vi "QT_MovieNew.vi"(1 "File Settings":T1 {"Dialogs" format="%.0b"}, 2 "Movie Settings":T4 {"Dialogs" format="%.0b"}, 3 "Compression Settings":T3 {"Dialogs" format="%.0b"; "Comp. Quality" format="%.0x"; "Codec" format="%.0x"}, 5 "error in (no error)":errorcluster, 8 "Private":T5, 9 "Transformation matrix":T2 {"Matrix" format="%.2f"}) -> (14 "QT Ref Out":T6, 19 "error out":errorcluster)   [LabVIEW 2024]
doc: "Create and initilize a new Frame grabber channel"
uses:
  <userlib>/ImageProcessing/QTLIB_2595_LV86/QT_Selector.ctl
  <userlib>/ImageProcessing/QTLIB_2595_LV86/QT_Ref.ctl
  <userlib>/ImageProcessing/QTLIB_2595_LV86/QT_Private.ctl
  <userlib>/ImageProcessing/QTLIB_2595_LV86/QT_Movie.ctl
  <userlib>/ImageProcessing/QTLIB_2595_LV86/QT_Compression.ctl
  <userlib>/ImageProcessing/QTLIB_2595_LV86/QT_File.ctl
  <userlib>/ImageProcessing/QTLIB_2595_LV86/QT_Effect.ctl
panel:
  # "[0,0] [0,1]  [0,2] [1,0].. [2,2]"
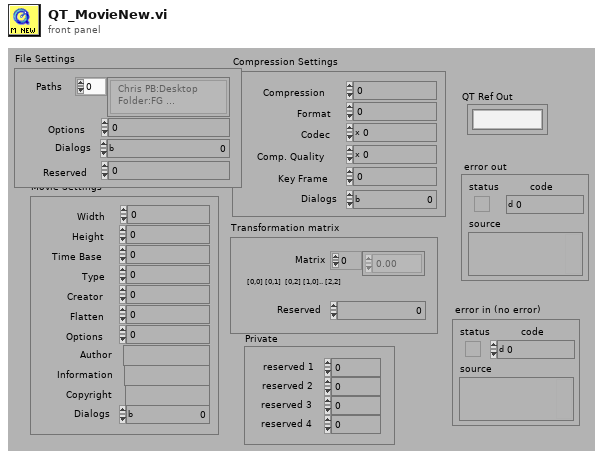
[diagram p1: front panel]
types:
  T1 = typedef "QT_File.ctl" = cluster{"Paths":string[], "Options":i32, "Dialogs":u32, "Reserved":i32}
  T2 = typedef "QT_Effect.ctl" = cluster{"Reserved":i32, "Matrix":dbl[]}
  T3 = typedef "QT_Compression.ctl" = cluster{"Compression":i32, "Format":i32, "Codec":i32, "Comp. Quality":i32, "Key Frame":i32, "Dialogs":u32}
  T4 = typedef "QT_Movie.ctl" = cluster{"Width":i32, "Height":i32, "Time Base":i32, "Type":i32, "Creator":i32, "Flatten":i32, "Options":i32, "Author":string, "Information":string, "Copyright":string, "Dialogs":u32}
  T5 = typedef "QT_Private.ctl" = cluster{"reserved 1":i32, "reserved 2":i32, "reserved 3":i32, "reserved 4":i32}
  T6 = typedef "QT_Ref.ctl" = refnum<k1>
  T7 = typedef "QT_Selector.ctl" = enum32{"do nothing", "Get all Sources", "Get Source info", "Open Image", "Save Image to File", "Effect", "Close", "SG Grab", "Compress in Memory", "Decompress to Memory", "New Movie", "Open Movie", "Add Frame", "Get Frame", "Close Movie", "Get QT & CIN info", "SG init", "SG Close", "Open sound file", "Close sound file", "Read sound data", "Write sound data", "Import sound", "Export sound", "Add sound to movie", "Get sound from movie", "reserved", "reserved 1", "reserved 2"}
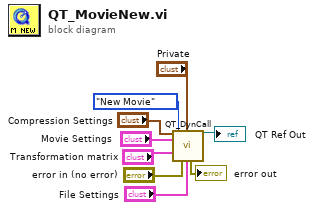
[diagram p0: block diagram]
diagram:
  n1 = call <userlib>:"QT_DynCall.vi"("Compression Settings"="Compression Settings", "Movie Settings"="Movie Settings", "error in (no error)"="error in (no error)", "Selector"=QT_Selector."New Movie", "Private"="Private", "Effect"="Transformation matrix", "File Settings"="File Settings") -> ("QT Ref Out"=→"QT Ref Out":T6, "error out"=→"error out":errorcluster)  [unwired: 5 in, 14 out]
